vi "InsertVI.vi"(8 "error in (no error)":errorcluster, 10 "VIPath":path, 11 "TabControl in":refnum<vi>) -> (0 "error out":errorcluster)   [LabVIEW 2020, in "MDI ViewManager.lvlib"]
uses:
  MDI ViewManager.lvlib
  <userlib>/_NEVSTOP/Communicable State Machine(CSM)/Communicable State Machine.lvlib
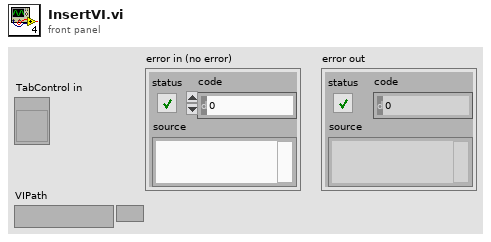
[diagram p1: front panel]
types:
  T1 = enum32{"Invalid", "Standard", "Closed", "Hidden", "Minimized", "Maximized"}
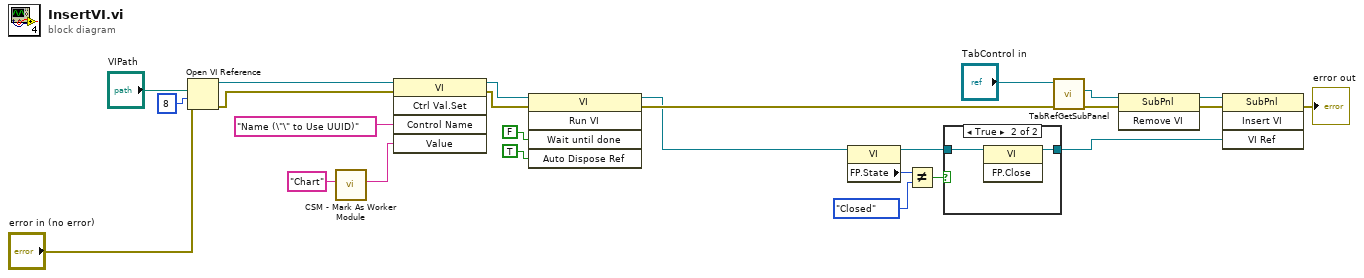
[diagram p0: block diagram]
diagram:
  n1 = Open VI Reference(vi path="VIPath", options=8, error in (no error)="error in (no error)") -> (vi reference=w20:refnum<vi>, error out=w6:errorcluster)  [unwired: 3 in]
  n2 = call <userlib>:"CSM - Mark As Worker Module.vi"("CSM Name"="Chart") -> ("CSM Name (Marked As Worker)"=w7:string)  [unwired: 9 in]
  n3 = invoke class="VI" method="Ctrl Val.Set"(reference=w20, error in=w6, "Control Name"="Name (\"\" to Use UUID)", "Value"=w7) -> (reference out=w9:refnum<vi>, error out=w5:errorcluster)  [unwired: 1 in, 3 out]
  n4 = invoke class="VI" method="Run VI"(reference=w9, error in=w5, "Wait until done"=FALSE ("Wait Until Done"), "Auto Dispose Ref"=TRUE ("Auto Dispose Reference")) -> (reference out=w17:refnum<vi>, error out=w25:errorcluster)  [unwired: 1 in, 3 out]
  n5 = property class="VI"(reference=w17) -> (reference out=w13:refnum<vi>, "FP.State"=w16:T1)  [unwired: 1 in, 1 out]
  n6 = Not Equal?(x=w16, y=T1."Closed") -> (x != y?=w14:bool)
  n7 = case shown="True" w14 {
    tunnel: w13 -> [w26 w28]
    tunnel: [w26 w27] -> w12
    frame False {
    }
    frame True {
      n8 = invoke class="VI" method="FP.Close"(reference=w28) -> (reference out=w27:refnum<vi>)  [unwired: 2 in, 2 out]
    }
  }
  n9 = call "TabRefGetSubPanel.vi"("error in (no error)"=w25, "TabControl in"="TabControl in") -> ("error out"=w4:errorcluster, "Sub Panel"=w22:refnum<vi>)  [unwired: 7 in, 1 out]
  n10 = invoke class="SubPnl" method="Remove VI"(reference=w22, error in=w4) -> (reference out=w11:refnum<vi>, error out=w3:errorcluster)  [unwired: 1 in, 1 out]
  n11 = invoke class="SubPnl" method="Insert VI"(reference=w11, error in=w3, "VI Ref"=w12) -> (error out=→"error out":errorcluster)  [unwired: 1 in, 3 out]
